vi "DSF.Engine.Plugin.Get Interface.vi"(11 "Plugin in":refnum<class "Plugin.lvclass">) -> (2 "Interface":refnum<class "DSF.Engine.Interface.Plugin.lvclass">, 3 "Plugin out":refnum<class "Plugin.lvclass">)   [LabVIEW 2017, in "DSF.Engine.lvlib" / "Plugin.lvclass"]
uses:
  Plugin.lvclass
  Interface/DSF.Engine.Interface.Plugin.lvclass
  Plugin.lvclass/Plugin.ctl
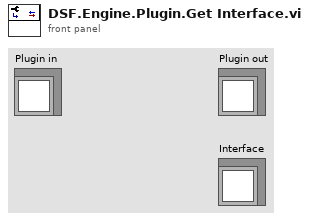
[diagram p1: front panel]
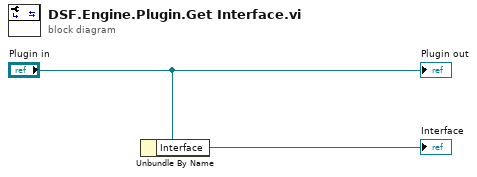
[diagram p0: block diagram]
diagram:
  n1 = Unbundle By Name("Plugin in") -> ("Interface"=→"Interface":refnum<class "DSF.Engine.Interface.Plugin.lvclass">)
  "Plugin out" <- "Plugin in"
